vi "AcquireHardware.vi"(8 "error in (no error)":errorcluster, 10 "Axis 1":string, 11 "NewportXPS in":refnum<class "NewportXPS.lvclass">) -> (0 "error out":errorcluster, 3 "Current position (units)":dbl)   [LabVIEW 2020, in "NewportXPS.lvclass"]
uses:
  NewportXPS.lvclass
  NewportXPS.lvclass/NewportXPS.ctl
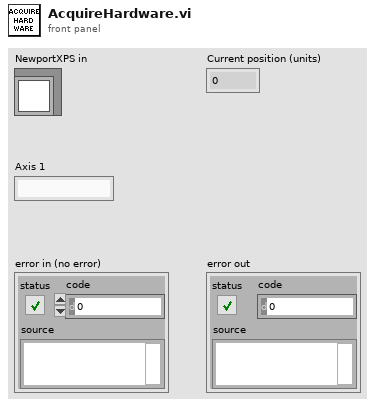
[diagram p1: front panel]
types:
  T1 = cluster{"connection TCP":refnum<k5>, "LogTo File":bool, "Log File refnum":refnum<file>, "no error if error log":bool}
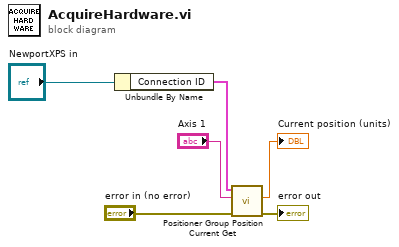
[diagram p0: block diagram]
diagram:
  n1 = Unbundle By Name("NewportXPS in") -> ("Connection ID"=w6:T1)
  n2 = call "Positioner Group Position Current Get.vi"("error in (no error)"="error in (no error)", "Positioner Name (250 c max)"="Axis 1", "connection ID in"=w6) -> ("error out"=→"error out":errorcluster, "Current position (units)"=→"Current position (units)":dbl)  [unwired: 5 in, 2 out]
